vi "Translator.File.Find.vi"(8 "error in":errorcluster, 11 "Translation folder":path=path "D:/PL_0125_Sapphire_Automation/settings") -> (0 "error out":errorcluster, 2 "Languages":string[](array[string]))   [LabVIEW 2019, in "Tools.lvlib"]
uses:
  Tools.lvlib
  Translator.Enums.ctl
  Translator.Global.vi
panel:
  in  "Enums":T1
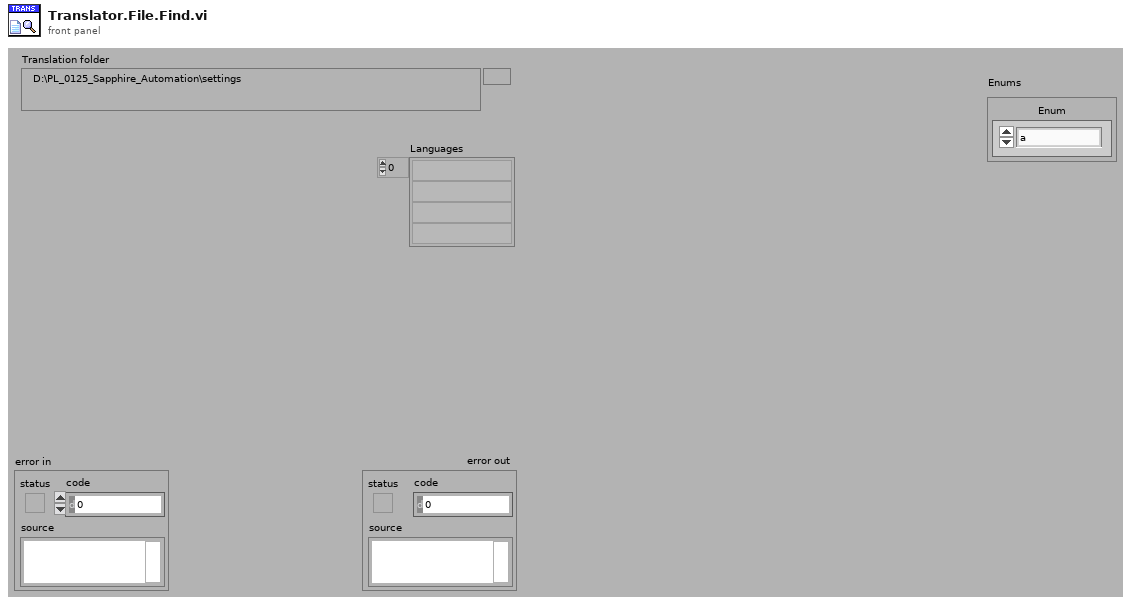
[diagram p1: front panel]
types:
  T1 = typedef "Tools.lvlib/Translator.Enums.ctl" = cluster{"Enum":enum16{"a", "b", "c"}}
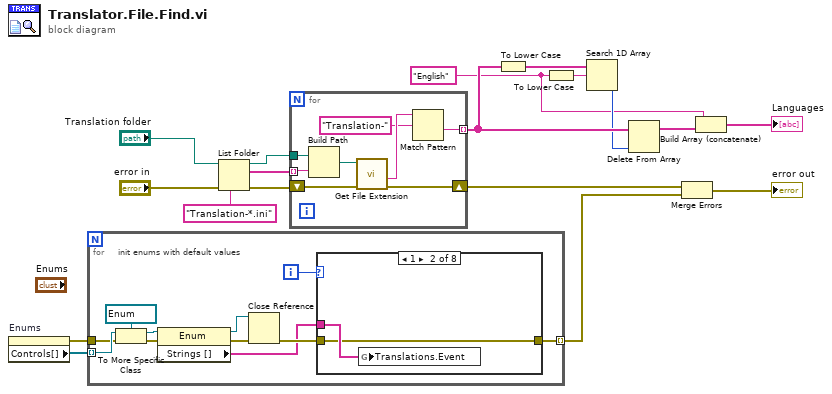
[diagram p0: block diagram]
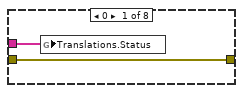
[diagram p2: hidden frame]
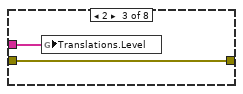
[diagram p3: hidden frame]
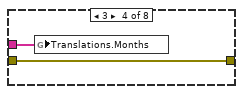
[diagram p4: hidden frame]
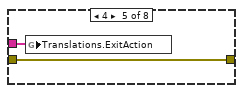
[diagram p5: hidden frame]
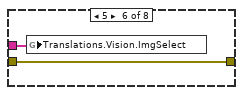
[diagram p6: hidden frame]
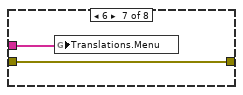
[diagram p7: hidden frame]
diagram:
  w5 = "English" ("element")
  n1 = property on="Enums" class="Clust (strict)"() -> (error out=w3:errorcluster, "Controls[]"=w4:refnum<vi>[])  [unwired: 2 in, 1 out]
  n2 = for {
    tunnel: w4 -> [w29] mode=indexing
    tunnel: w3 -> [w25]
    tunnel: [w22] -> w1 mode=indexing
    i -> [w19]
    # "init enums with default values"
    n3 = To More Specific Class(target class=refnum<vi> refnum ("reference out"), reference=w29, error in=w25) -> (specific class reference=w28:refnum<vi>, error out=w27:errorcluster)
    n4 = property class="Enum"(reference=w28, error in=w27) -> (reference out=w23:refnum<vi>, error out=w24:errorcluster, "Strings []"=w20:string[])
    n5 = Close Reference(reference=w23, error in (no error)=w24) -> (error out=w21:errorcluster)
    n6 = case shown="1" w19 {
      tunnel: w20 -> [w31 w33 w35 w37 w39 w41 w43 _]
      tunnel: w21 -> [w30 w32 w34 w36 w38 w40 w42 w44]
      tunnel: [w30 w32 w34 w36 w38 w40 w42 w44] -> w22
      frame 0 {
        n7 = global write "Translator.Global.vi" "Translations.Status"(w31) -> ()
      }
      frame 1 {
        n8 = global write "Translator.Global.vi" "Translations.Event"(w33) -> ()
      }
      frame 2 {
        n9 = global write "Translator.Global.vi" "Translations.Level"(w35) -> ()
      }
      frame 3 {
        n10 = global write "Translator.Global.vi" "Translations.Months"(w37) -> ()
      }
      frame 4 {
        n11 = global write "Translator.Global.vi" "Translations.ExitAction"(w39) -> ()
      }
      frame 5 {
        n12 = global write "Translator.Global.vi" "Translations.Vision.ImgSelect"(w41) -> ()
      }
      frame 6 {
        n13 = global write "Translator.Global.vi" "Translations.Menu"(w43) -> ()
      }
      frame Default {
      }
    }
  }
  n14 = List Folder(path="Translation folder", pattern="Translation-*.ini", error in="error in") -> (path out=w11:path, filenames=w12:string[], error out=w13:errorcluster)  [unwired: 1 in, 1 out]
  n15 = for {
    tunnel: w12 -> [w51] mode=indexing
    tunnel: w11 -> [w52]
    tunnel: [w45] -> w9 mode=indexing
    shift-right: [w48] -> w17
    shift-left: w13 -> [w49]
    n16 = Build Path(base path=w52, name or relative path=w51) -> (appended path=w50:path)
    n17 = call <vilib>:"Get File Extension.vi"("error in (no error)"=w49, "file"=w50) -> ("error out"=w48:errorcluster, "filename without extension"=w47:string)  [unwired: 5 in, 3 out]
    n18 = Match Pattern(string=w47, regular expression="Translation-" ("pattern")) -> (after substring=w45:string)  [unwired: 1 in, 3 out]
  }
  n19 = To Lower Case(string=w9) -> (all lower case string=w10:string[])
  n20 = To Lower Case(string=w5) -> (all lower case string=w6:string)
  n21 = Search 1D Array(1D array=w10, element=w6) -> (index of element=w7:i32)  [unwired: 1 in]
  n22 = Delete From Array(array=w9, index=w7) -> (array with subset deleted=w8:string[])  [unwired: 1 in, 1 out]
  n23 = Merge Errors(w17, w1) -> (→"error out":errorcluster)
  n24 = Build Array (concatenate)(w5, w8) -> (→"Languages":string[])
